vi "Wyznaczenie formatu wprowadzonej współrzędnej.vi"(10 "Współrzędna geograficzna":string) -> (0 "error constant":errorcluster, 1 "Format wprowadzonej współrzędnej":i32, 2 "Znaleziony tekst":string)   [LabVIEW 2012, in "Biblioteka moduł map v3.lvlib" / "Konwersja wsp.lvlib" / "Wyciągnięcie z tekstu współrzędnej.lvlib"]
doc: "SubVI przeszukuje wpisany tekst w poszukiwaniu znanych mu formatów współrzędnych punktu. Jeżeli format został rozpoznany zwracana jest wartość współrzędnej w formacie tekstowym. W przypadku błędu nie zostanie odnaleziony, żeden tekst."
panel:
  in  "Wzory wprowadzanych współrzędnych":u16(ring) items=["D (długość, szerokość)", "D (szerokość, długość)", "DM (długość, szerokość)", "DM (szerokość, długość)", "DMS (długość, szerokość)", "DMS (szerokość, długość)"]
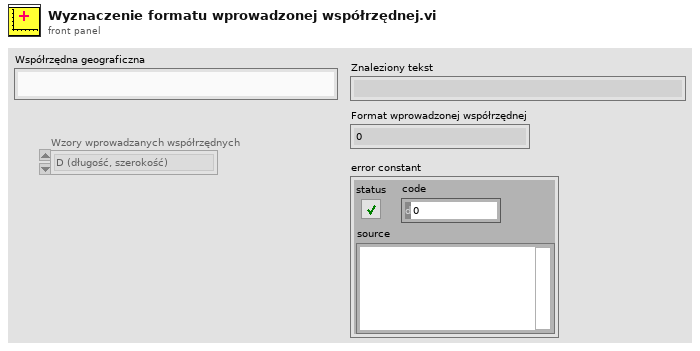
[diagram p1: front panel]
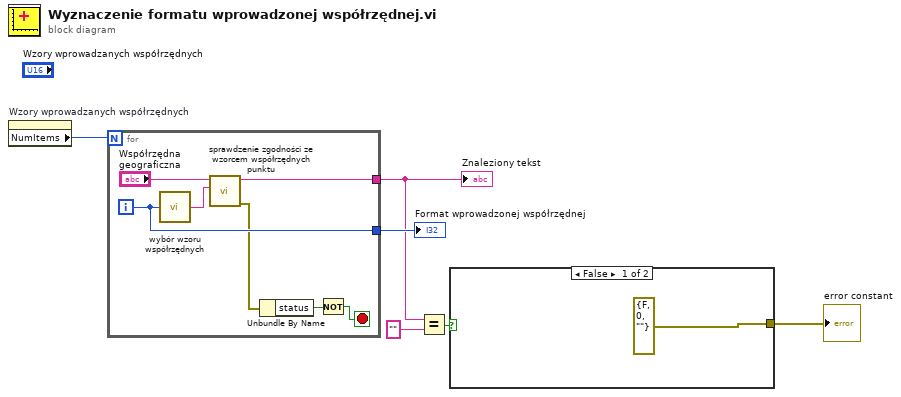
[diagram p0: block diagram]
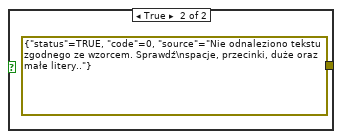
[diagram p2: hidden frame]
diagram:
  n1 = property on="Wzory wprowadzanych współrzędnych" class="Ring (strict)"() -> ("NumItems"=w6:u32)  [unwired: 2 in, 2 out]
  n2 = for {
    N: w6 -> [_]
    tunnel: [w12] -> w3
    tunnel: [w11] -> w5
    i -> [w11]
    stop <- w7 stop-if-true
    n3 = call "wybór wzoru współrzędnych.vi"("Wzory wprowadzanych współrzędnych"=w11) -> ("Wzór szukanych współrzędnych punktu"=w9:string)  [unwired: 4 in]
    n4 = call "sprawdzenie zgodności ze wzorcem współrzędnych punktu.vi"("Tekst"="Współrzędna geograficzna", "Wzór"=w9) -> ("Znaleziony tekst"=w12:string, "Nieprawidłowy wzór"=w10:errorcluster)  [unwired: 7 in]
    n5 = Unbundle By Name(w10) -> ("status"=w8:bool)
    n6 = Not(x=w8) -> (.not. x?=w7:bool)
  }
  "Znaleziony tekst" <- w3
  "Format wprowadzonej współrzędnej" <- w5
  n7 = Equal?(x=w3, y="") -> (x = y?=w4:bool)
  n8 = case shown="False" w4 {
    tunnel: [errorcluster {"status"=FALSE, "code"=0, "source"=""} ("error constant") errorcluster {"status"=TRUE, "code"=0, "source"="Nie odnaleziono tekstu zgodnego ze wzorcem. Sprawdź\nspacje, przecinki, duże oraz małe litery.."} ("error constant")] -> w1
    frame False {
    }
    frame True {
    }
  }
  "error constant" <- w1
